vi "Menu Property Item to Query.vi"(8 "error in (no error)":errorcluster, 10 "Custom Search Parameters":T5, 11 "Connection Refnum In":T1) -> (0 "error out":errorcluster, 1 "Query Summary":string, 2 "Custom Search Parameters":T2[](array[typedef]), 3 "Connection Refnum Out":T1)   [LabVIEW 2011]
uses:
  Query Parameters.ctl
  DataFinder/Datafinder Query.ctl
  DataFinder/eSearch Types.ctl
  DataFinder/DataFinder Comparisons.ctl
  SI.LIB/ODBC/SQL Controls/Connection Refnum.ctl
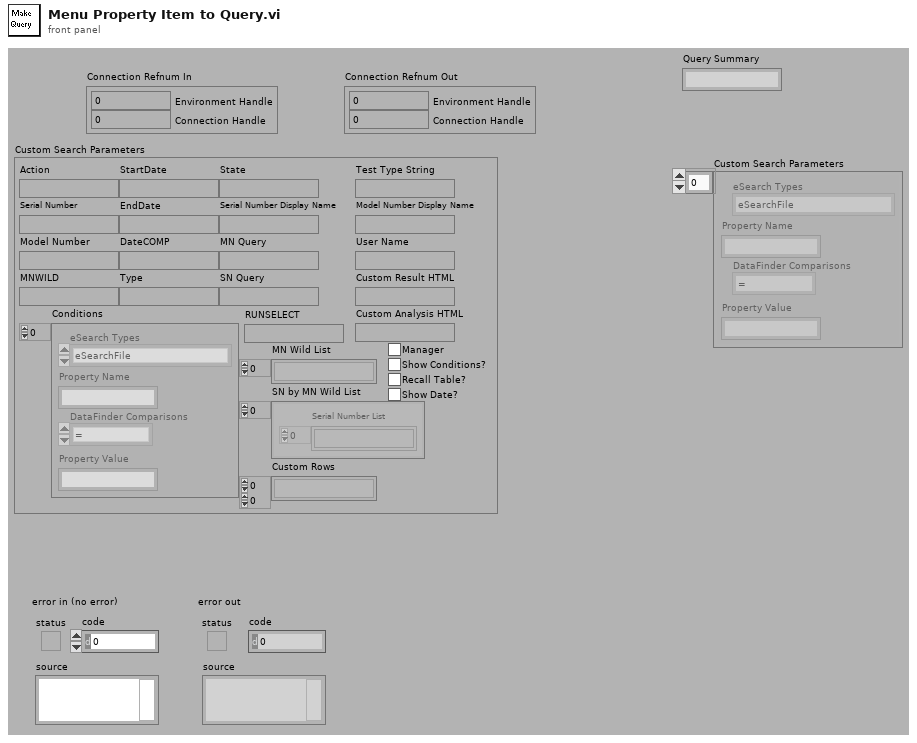
[diagram p1: front panel]
types:
  T1 = typedef "Connection Refnum.ctl" = cluster{"Environment Handle":i32, "Connection Handle":i32}
  T2 = typedef "Datafinder Query.ctl" = cluster{"eSearch Types":T3, "Property Name":string, "DataFinder Comparisons":T4, "Property Value":string}
  T3 = typedef "eSearch Types.ctl" = enum16{"eSearchFile", "eSearchChannelGroup", "eSearchChannel"}
  T4 = typedef "DataFinder Comparisons.ctl" = enum16{"=", "<>", "<", "<=", ">", ">="}
  T5 = typedef "Query Parameters.ctl" = cluster{"Action":string, "Serial Number":string, "Model Number":string, "MNWILD":string, "StartDate":string, "EndDate":string, "DateCOMP":string, "Conditions":T2[], "MN Wild List":string[], "SN by MN Wild List":cluster{"Serial Number List":string[]}[], "Recall Table?":bool, "Type":string, "Show Date?":bool, "Show Conditions?":bool, "Serial Number Display Name":string, "Model Number Display Name":string, "Test Type String":string, "Manager":bool, "Custom Rows":string[][], "Custom Result HTML":string, "User Name":string, "State":string, "MN Query ":string, "SN Query":string, "Custom Analysis HTML":string, "RUNSELECT":string}
  T6 = typedef "LVDateTimeRec.ctl" = cluster{"fractional second":dbl, "second":i32, "minute":i32, "hour":i32, "day of month":i32, "month":i32, "year":i32, "day of week":i32, "day of year":i32, "DST":i32}
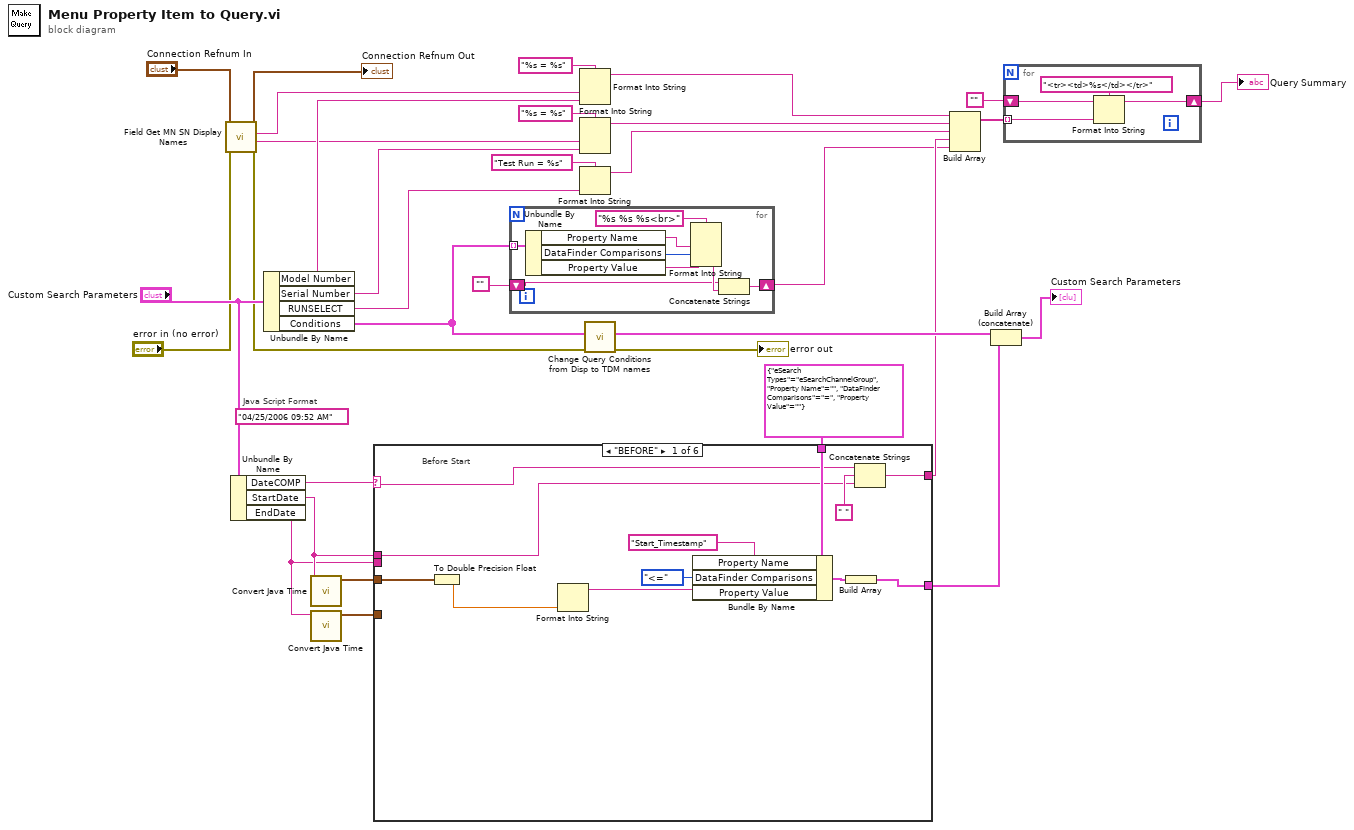
[diagram p0: block diagram]
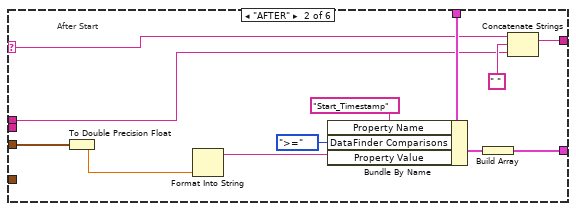
[diagram p2: hidden frame]
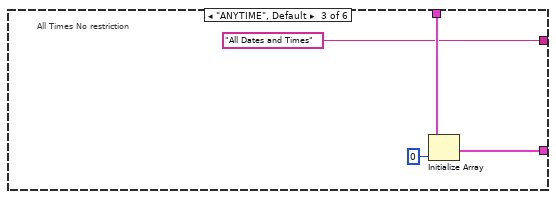
[diagram p3: hidden frame]
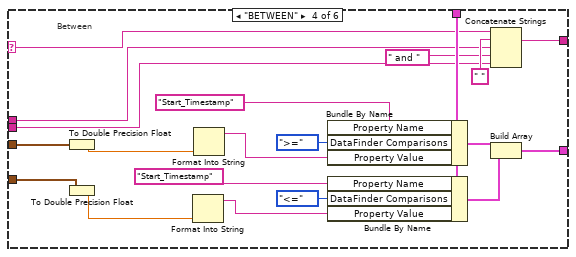
[diagram p4: hidden frame]
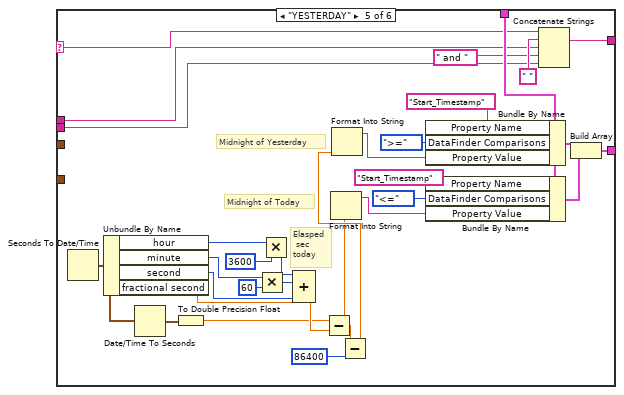
[diagram p5: hidden frame]
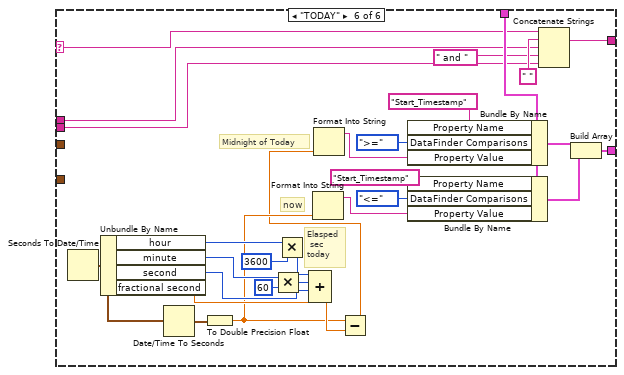
[diagram p6: hidden frame]
diagram:
  (unwired) "04/25/2006 09:52 AM" ("key")
  # "Java Script Format"
  n1 = call "Field Get MN SN Display Names.vi"("error in (no error)"="error in (no error)", "Connection Refnum"="Connection Refnum In") -> ("error out"=w21:errorcluster, "Serial Number Display Name"=w17:string, "Model Number Display Name"=w20:string, "Connection Refnum"=→"Connection Refnum Out":T1)  [unwired: 6 out]
  n2 = Unbundle By Name("Custom Search Parameters") -> ("DateCOMP"=w27:string, "StartDate"=w11:string, "EndDate"=w10:string)
  n3 = Unbundle By Name("Custom Search Parameters") -> ("Model Number"=w19:string, "Serial Number"=w16:string, "RUNSELECT"=w7:string, "Conditions"=w14:T2[])
  n4 = call "Convert Java Time.vi"("Date/Time"=w11) -> ("Time Stamp"=w25:timestamp)  [unwired: 10 out]
  n5 = call "Convert Java Time.vi"("Date/Time"=w10) -> ("Time Stamp"=w26:timestamp)  [unwired: 10 out]
  n6 = case shown="\"BEFORE\"" w27 {
    selector: w27 -> [w35 w47 _ w66 w101 w130]
    tunnel: w25 -> [w45 w57 _ w81 _ _]
    tunnel: w26 -> [_ _ _ w75 _ _]
    tunnel: T2 {"eSearch Types"=enum."eSearchChannelGroup", "Property Name"="", "DataFinder Comparisons"=enum."=", "Property Value"=""} ("Data Finder Parameters") -> [w40 w50 w61 w69 w104 w133]
    tunnel: [w38 w51 w59 w68 w103 w132] -> w29
    tunnel: [w36 w48 "All Dates and Times" ("format string") w67 w102 w131] -> w12
    tunnel: w11 -> [w34 w46 _ w64 w99 w128]
    tunnel: w10 -> [_ _ _ w62 w97 w126]
    frame "BEFORE" {
      # "Before Start"
      n7 = To Double Precision Float(number=w45) -> (double precision float=w42:dbl)
      n8 = Format Into String(w42) -> (resulting string=w41:string)  [unwired: 3 in, 1 out]
      n9 = Bundle By Name(cluster=w40, "Property Name"="Start_Timestamp", "DataFinder Comparisons"=DataFinder_Comparisons."<=", "Property Value"=w41) -> (w39:T2)
      n10 = Build Array(w39) -> (w38:T2[])
      n11 = Concatenate Strings(w35, " " ("format string"), w34) -> (w36:string)
    }
    frame "AFTER" {
      # "After Start"
      n12 = To Double Precision Float(number=w57) -> (double precision float=w54:dbl)
      n13 = Format Into String(w54) -> (resulting string=w53:string)  [unwired: 3 in, 1 out]
      n14 = Bundle By Name(cluster=w50, "Property Name"="Start_Timestamp", "DataFinder Comparisons"=DataFinder_Comparisons.">=", "Property Value"=w53) -> (w52:T2)
      n15 = Build Array(w52) -> (w51:T2[])
      n16 = Concatenate Strings(w47, " " ("format string"), w46) -> (w48:string)
    }
    frame "ANYTIME", Default {
      # "All Times No restriction"
      n17 = Initialize Array(w61, 0 ("dimension size")) -> (w59:T2[])
    }
    frame "BETWEEN" {
      # "Between"
      n18 = To Double Precision Float(number=w81) -> (double precision float=w79:dbl)
      n19 = To Double Precision Float(number=w75) -> (double precision float=w74:dbl)
      n20 = Format Into String(w74) -> (resulting string=w73:string)  [unwired: 3 in, 1 out]
      n21 = Format Into String(w79) -> (resulting string=w78:string)  [unwired: 3 in, 1 out]
      n22 = Bundle By Name(cluster=w69, "Property Name"="Start_Timestamp", "DataFinder Comparisons"=DataFinder_Comparisons.">=", "Property Value"=w78) -> (w71:T2)
      n23 = Bundle By Name(cluster=w69, "Property Name"="Start_Timestamp", "DataFinder Comparisons"=DataFinder_Comparisons."<=", "Property Value"=w73) -> (w70:T2)
      n24 = Concatenate Strings(w66, " " ("format string"), w64, " and " ("format string"), w62) -> (w67:string)
      n25 = Build Array(w71, w70) -> (w68:T2[])
    }
    frame "YESTERDAY" {
      # "Elasped\n sec\ntoday"
      # "Midnight of Yesterday"
      # "Midnight of Today"
      n26 = Seconds To Date/Time() -> (date time rec=w92:T6)  [unwired: 2 out]
      n27 = Unbundle By Name(w92) -> ("hour"=w84:i32, "minute"=w87:i32, "second"=w86:i32, "fractional second"=w85:dbl)
      n28 = Date/Time To Seconds(2:w92) -> (0:w93:timestamp)  [unwired: 1 out]
      n29 = To Double Precision Float(number=w93) -> (double precision float=w94:dbl)
      n30 = Multiply(x=w87, y=60) -> (x*y=w89:i32)
      n31 = Multiply(x=w84, y=3600) -> (x*y=w91:i32)
      n32 = Compound Arithmetic op=ADD(w91, w89, w86, w85) -> (w95:dbl)
      n33 = Subtract(x=w94, y=w95) -> (x-y=w82:dbl)
      n34 = Format Into String(w82) -> (resulting string=w108:string)  [unwired: 3 in, 1 out]
      n35 = Subtract(x=w82, y=86400) -> (x-y=w83:dbl)
      n36 = Format Into String(w83) -> (resulting string=w111:string)  [unwired: 3 in, 1 out]
      n37 = Bundle By Name(cluster=w104, "Property Name"="Start_Timestamp", "DataFinder Comparisons"=DataFinder_Comparisons.">=", "Property Value"=w111) -> (w106:T2)
      n38 = Bundle By Name(cluster=w104, "Property Name"="Start_Timestamp", "DataFinder Comparisons"=DataFinder_Comparisons."<=", "Property Value"=w108) -> (w105:T2)
      n39 = Concatenate Strings(w101, " " ("format string"), w99, " and " ("format string"), w97) -> (w102:string)
      n40 = Build Array(w106, w105) -> (w103:T2[])
    }
    frame "TODAY" {
      # "Elasped\n sec\ntoday"
      # "Midnight of Today"
      # "now"
      n41 = Seconds To Date/Time() -> (date time rec=w123:T6)  [unwired: 2 out]
      n42 = Unbundle By Name(w123) -> ("hour"=w115:i32, "minute"=w118:i32, "second"=w117:i32, "fractional second"=w116:dbl)
      n43 = Date/Time To Seconds(2:w123) -> (0:w124:timestamp)  [unwired: 1 out]
      n44 = To Double Precision Float(number=w124) -> (double precision float=w114:dbl)
      n45 = Multiply(x=w118, y=60) -> (x*y=w120:i32)
      n46 = Multiply(x=w115, y=3600) -> (x*y=w122:i32)
      n47 = Compound Arithmetic op=ADD(w122, w120, w117, w116) -> (w125:dbl)
      n48 = Format Into String(w114) -> (resulting string=w137:string)  [unwired: 3 in, 1 out]
      n49 = Subtract(x=w114, y=w125) -> (x-y=w113:dbl)
      n50 = Format Into String(w113) -> (resulting string=w140:string)  [unwired: 3 in, 1 out]
      n51 = Bundle By Name(cluster=w133, "Property Name"="Start_Timestamp", "DataFinder Comparisons"=DataFinder_Comparisons.">=", "Property Value"=w140) -> (w135:T2)
      n52 = Bundle By Name(cluster=w133, "Property Name"="Start_Timestamp", "DataFinder Comparisons"=DataFinder_Comparisons."<=", "Property Value"=w137) -> (w134:T2)
      n53 = Concatenate Strings(w130, " " ("format string"), w128, " and " ("format string"), w126) -> (w131:string)
      n54 = Build Array(w135, w134) -> (w132:T2[])
    }
  }
  n55 = for {
    shift-right: [w142] -> w9
    shift-left: "" -> [w143]
    tunnel: w14 -> [w148] mode=indexing
    n56 = Unbundle By Name(w148) -> ("Property Name"=w147:string, "DataFinder Comparisons"=w146:T4, "Property Value"=w145:string)
    n57 = Format Into String(format string="%s %s %s<br>", w147, w146, w145) -> (resulting string=w144:string)  [unwired: 2 in, 1 out]
    n58 = Concatenate Strings(w143, w144) -> (w142:string)
  }
  n59 = Format Into String(format string="%s = %s", w20, w19) -> (resulting string=w23:string)  [unwired: 2 in, 1 out]
  n60 = Format Into String(format string="%s = %s", w17, w16) -> (resulting string=w13:string)  [unwired: 2 in, 1 out]
  n61 = Format Into String(format string="Test Run = %s", w7) -> (resulting string=w6:string)  [unwired: 2 in, 1 out]
  n62 = call "Change Query Conditions from Disp to TDM names.vi"("error in (no error)"=w21, "Conditions"=w14) -> ("error out"=→"error out":errorcluster, "Array"=w30:T2[])  [unwired: 1 in, 7 out]
  n63 = Build Array(w23, w13, w6, w12, w9) -> (w4:string[])
  n64 = Build Array (concatenate)(w30, w29) -> (→"Custom Search Parameters":T2[])
  n65 = for {
    shift-right: [w152] -> w3
    shift-left: "" -> [w153]
    tunnel: w4 -> [w150] mode=indexing
    n66 = Format Into String(format string="<tr><td>%s</td></tr>", initial string=w153, w150) -> (resulting string=w152:string)  [unwired: 1 in, 1 out]
  }
  "Query Summary" <- w3
